vi "Drive.vi"(8 "error in (no error)":errorcluster) -> ()   [LabVIEW 2014]
uses:
  <vilib>/Rock Robotics/WPI/RobotDrive/WPI_RobotDriveGetSetRefNum.vi
  Robot Global Data.vi
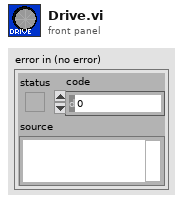
[diagram p1: front panel]
types:
  T1 = typedef "WPI_RobotDriveDevRef.ctl" = cluster{"DevStatus":errorcluster, "Motors[]":T2[], "Square Inputs":bool, "Max Output":dbl}
  T2 = typedef "WPI_MotorControlDeviceRef.ctl" = cluster{"DeviceStatus":errorcluster, "Type":enum16{"PWM", "CAN"}, "PWM":cluster{"Digital Module":T3, "PWM Channel":T4, "DeadBand":T5}, "CAN":cluster{"Device Number":u8, "Control Mode":T6, "Semaphore":T7, "Max Vout":dbl}, "Invert":bool, "TransformRef":T8, "InvTransformRef":T8}
  T3 = typedef "FPGA_TypedefDigitalModule.ctl" = enum16{"Digital Module 1", "Digital Module 2"}
  T4 = typedef "FPGA_DIOPWMChannel.ctl" = enum8{"PWM 1", "PWM 2", "PWM 3", "PWM 4", "PWM 5", "PWM 6", "PWM 7", "PWM 8", "PWM 9", "PWM 10", "Invalid"}
  T5 = typedef "WPI_PWMDeadband.ctl" = cluster{"Name":string, "maxPositivePwm":i32, "minPositivePwm":i32, "centerPwm":i32, "maxNegativePwm":i32, "minNegativePwm":i32, "angularRange":u16}
  T6 = typedef "WPI_CANJaguar_ControlMode.ctl" = enum8{"Percent VBus", "Current", "Speed", "Position", "Voltage"}
  T7 = typedef "Semaphore RefNum" = refnum<k1>
  T8 = typedef "WPI_PWMTransform_ConPane.ctl" = refnum<vi>
  T9 = typedef "User Commands typedef.ctl" = cluster{"Arm Command":T10, "Shooter Commands":T12, "Drive Commands":T13}
  T10 = typedef "Arm control typedef.ctl" = cluster{"Arm up/dwn":dbl, "Arm Capture":bool, "Arm Pass":bool, "Arm Positions":T11, "Arm Manual Override":bool}
  T11 = typedef "Arm Postions Enum Typedef.ctl" = enum16{"Arm Pick-up", "Idle", "Arm Shoot", "Arm Truss", "Manual"}
  T12 = typedef "Shooter Commands Typedef.ctl" = cluster{"Shooter Fire":bool, "Shooter Draw":bool}
  T13 = typedef "Drive Commands Typedef.ctl" = cluster{"Drive L/R":dbl, "Drive Fwd/Rev":dbl}
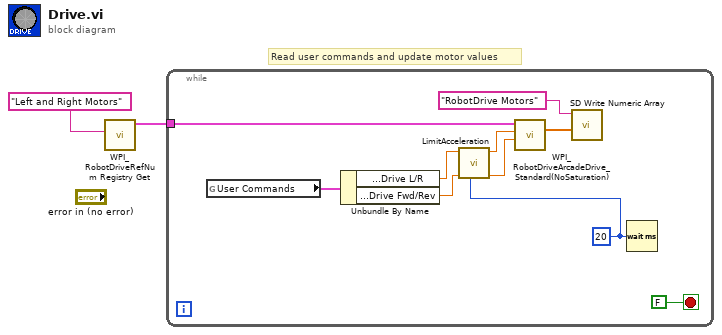
[diagram p0: block diagram]
diagram:
  # "Read user commands and update motor values"
  n1 = call <vilib>:"WPI_RobotDriveRefNum Registry Get.vi"("refnum name"="Left and Right Motors") -> ("RobotDriveDevRef"=w2:T1)  [unwired: 1 in, 9 out]
  n2 = while {
    tunnel: w2 -> [w8]
    stop <- FALSE stop-if-true
    w3 = u32 20 ("milliseconds to wait")
    n3 = global read "Robot Global Data.vi" "User Commands"() -> (w10:T9)
    n4 = Unbundle By Name(w10) -> ("Drive Commands.Drive L/R"=w7:dbl, "Drive Commands.Drive Fwd/Rev"=w6:dbl)
    n5 = call "LimitAcceleration.vi"("MsPerLoop"=w3, "YAxisIn"=w6, "XAxisIn"=w7) -> ("YAxisOut"=w4:dbl, "XAxisOut"=w5:dbl)  [unwired: 7 in]
    n6 = call <vilib>:"WPI_RobotDriveArcadeDrive_Standard(NoSaturation).vi"("Y axis value"=w4, "X axis value"=w5, "RobotDriveDevRef"=w8) -> ("Motor Values"=w12:dbl[])  [unwired: 1 in, 7 out]
    n7 = call <vilib>:"SD Write Numeric Array.vi"("Numeric Array"=w12, "Name"="RobotDrive Motors") -> ()  [unwired: 8 in, 2 out]
    n8 = Wait (ms)(milliseconds to wait=w3) -> ()  [unwired: 1 out]
  }
